vi "QTrkCUDA_QueryDevices.vi"(8 "error in (no error)":errorcluster) -> (0 "error out":errorcluster, 2 "number of CUDA devices":i32, 3 "CUDA devices":T1(array[cluster]))   [LabVIEW 2011]
uses:
  QTrkDLL.vi
panel:
  in  "CUDA Device":T2
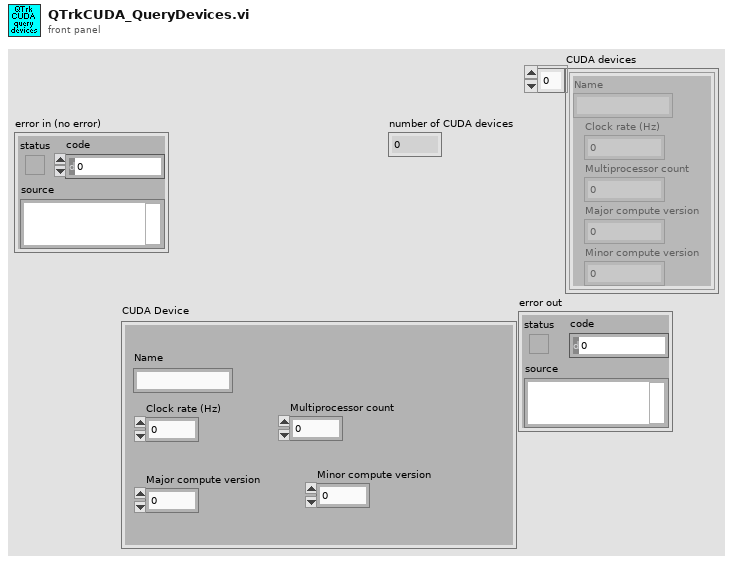
[diagram p1: front panel]
types:
  T1 = cluster{"Name":string, "Clock rate (Hz)":i32, "Multiprocessor count":i32, "Major compute version":i32, "Minor compute version":i32}[]
  T2 = cluster{"Name":string, "Clock rate (Hz)":i32, "Multiprocessor count":i32, "Major compute version":i32, "Minor compute version":i32}
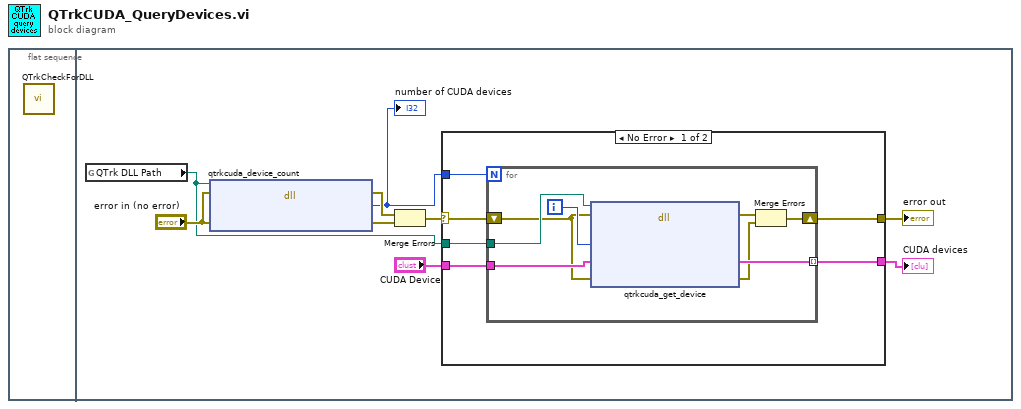
[diagram p0: block diagram]
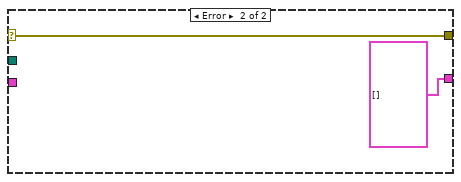
[diagram p2: hidden frame]
diagram:
  n1 = flat-sequence {
    frame #0 {
      n2 = call "QTrkCheckForDLL.vi"() -> ()  [unwired: 12 in]
    }
    frame #1 {
      n3 = global read "QTrkDLL.vi" "QTrk DLL Path"() -> (w5:path)
      n4 = dll-call lib="E:/Margreet/integrate camera into main program/jtrkcuda-labview.dll" fn="qtrkcuda_device_count"(path in=w5, error in="error in (no error)", "error"="error in (no error)") -> (error out=w9:errorcluster, "number of devices"=w3:i32, "error"=w7:errorcluster)  [unwired: 1 in, 1 out]
      "number of CUDA devices" <- w3
      n5 = Merge Errors(w9, w7) -> (w6:errorcluster)
      n6 = case shown="No Error" w6 {
        selector: w6 -> [w11 w25]
        tunnel: w3 -> [w15 _]
        tunnel: w5 -> [w14 _]
        tunnel: "CUDA Device" -> [w13 _]
        tunnel: [w12 T1 []] -> w1
        tunnel: [w10 w25] -> w2
        frame No Error {
          n7 = for {
            N: w15 -> [_]
            tunnel: w14 -> [w23]
            tunnel: w13 -> [w21]
            tunnel: [w20] -> w12 mode=indexing
            shift-right: [w17] -> w10
            shift-left: w11 -> [w16]
            i -> [w22]
            n8 = dll-call lib="E:/Margreet/integrate camera into main program/jtrkcuda-labview.dll" fn="qtrkcuda_get_device"(path in=w23, error in=w16, "device index"=w22, "device info"=w21, "error"=w16) -> (error out=w19:errorcluster, "device info"=w20:T2, "error"=w18:errorcluster)  [unwired: 3 in, 1 out]
            n9 = Merge Errors(w19, w18) -> (w17:errorcluster)
          }
        }
        frame Error {
        }
      }
      "CUDA devices" <- w1
      "error out" <- w2
    }
  }
